vi "Main - Update Tree (eFGV).vi"(7 "Action":T1, 8 "error in":errorcluster, 11 "Machine Table":string[][](array[string])) -> (0 "error out":errorcluster, 2 "Machine Ref":refnum<user-event>, 3 "Machine Table out":string[][](array[string]))   [LabVIEW 2019]
uses:
  Controls/eFGV States.ctl
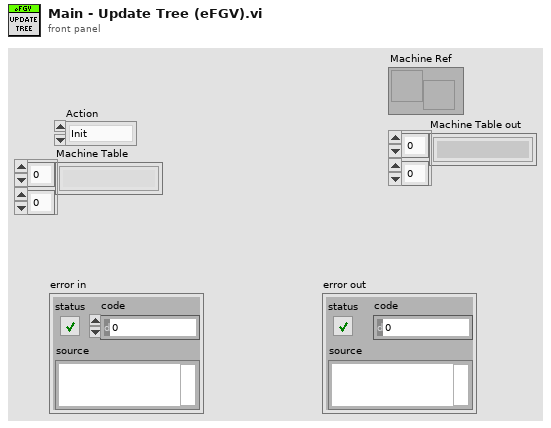
[diagram p1: front panel]
types:
  T1 = typedef "eFGV States.ctl" = enum16{"Init", "Read", "Write", "Exit"}
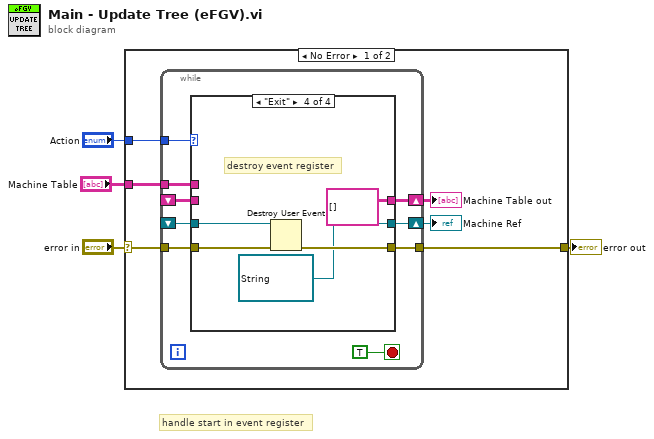
[diagram p0: block diagram]
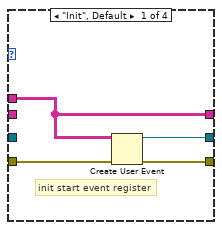
[diagram p2: hidden frame]
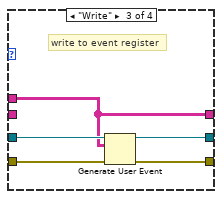
[diagram p4: hidden frame]
diagram:
  # "handle start in event register"
  n1 = case shown="No Error" "error in" {
    selector: "error in" -> [w8 w37]
    tunnel: "Action" -> [w10 _]
    tunnel: [w9 w37] -> w3
    tunnel: "Machine Table" -> [w7 _]
    frame No Error {
      n2 = while {
        tunnel: w10 -> [w18]
        tunnel: w8 -> [w17]
        tunnel: [w16] -> w9
        tunnel: w7 -> [w15]
        shift-right: [w14] -> w6
        shift-left: _ -> [w13]
        shift-right: [w12] -> w5
        shift-left: _ -> [w11]
        stop <- TRUE stop-if-true
        n3 = case shown="\"Exit\"" w18 {
          tunnel: w17 -> [w23 w26 w29 w36]
          tunnel: [w22 w26 w31 w35] -> w16
          tunnel: w13 -> [_ w25 w30 w34]
          tunnel: w15 -> [w20 _ w27 _]
          tunnel: [w21 w25 w28 refnum<user-event> refnum ("Machine Table")] -> w14
          tunnel: [w20 w24 w27 string[][] [] ("Machine Table")] -> w12
          tunnel: w11 -> [_ w24 _ _]
          frame "Init", Default {
            # "init start event register"
            n4 = Create User Event(user event datatype=w20, error in=w23) -> (user event=w21:refnum<user-event>, error out=w22:errorcluster)
          }
          frame "Read" {
            # "read from event register"
          }
          frame "Write" {
            # "write to event register"
            n5 = Generate User Event(user event=w30, event data cluster=w27, error in=w29) -> (user event out=w28:refnum<user-event>, error out=w31:errorcluster)  [unwired: 1 in]
          }
          frame "Exit" {
            # "destroy event register"
            n6 = Destroy User Event(user event=w34, error in=w36) -> (error out=w35:errorcluster)
          }
        }
      }
      "Machine Ref" <- w6
      "Machine Table out" <- w5
    }
    frame Error {
    }
  }
  "error out" <- w3
